vi "Sekvenser GFV.vi"(1 "Action(GET)":enum16{"GET", "SET"}(ring), 7 "Sequences":T1[](array[typedef]), 11 "error in (no error)":errorcluster) -> (8 "Sequences out":T1[](array[typedef]), 15 "error out":errorcluster)   [LabVIEW 2011]
uses:
  Complete sequence cluster holder.ctl
  User input.ctl
  Sequence steps config..ctl
  Single criteria cluster.ctl
  Criteria types.ctl
  Boolean operation.ctl
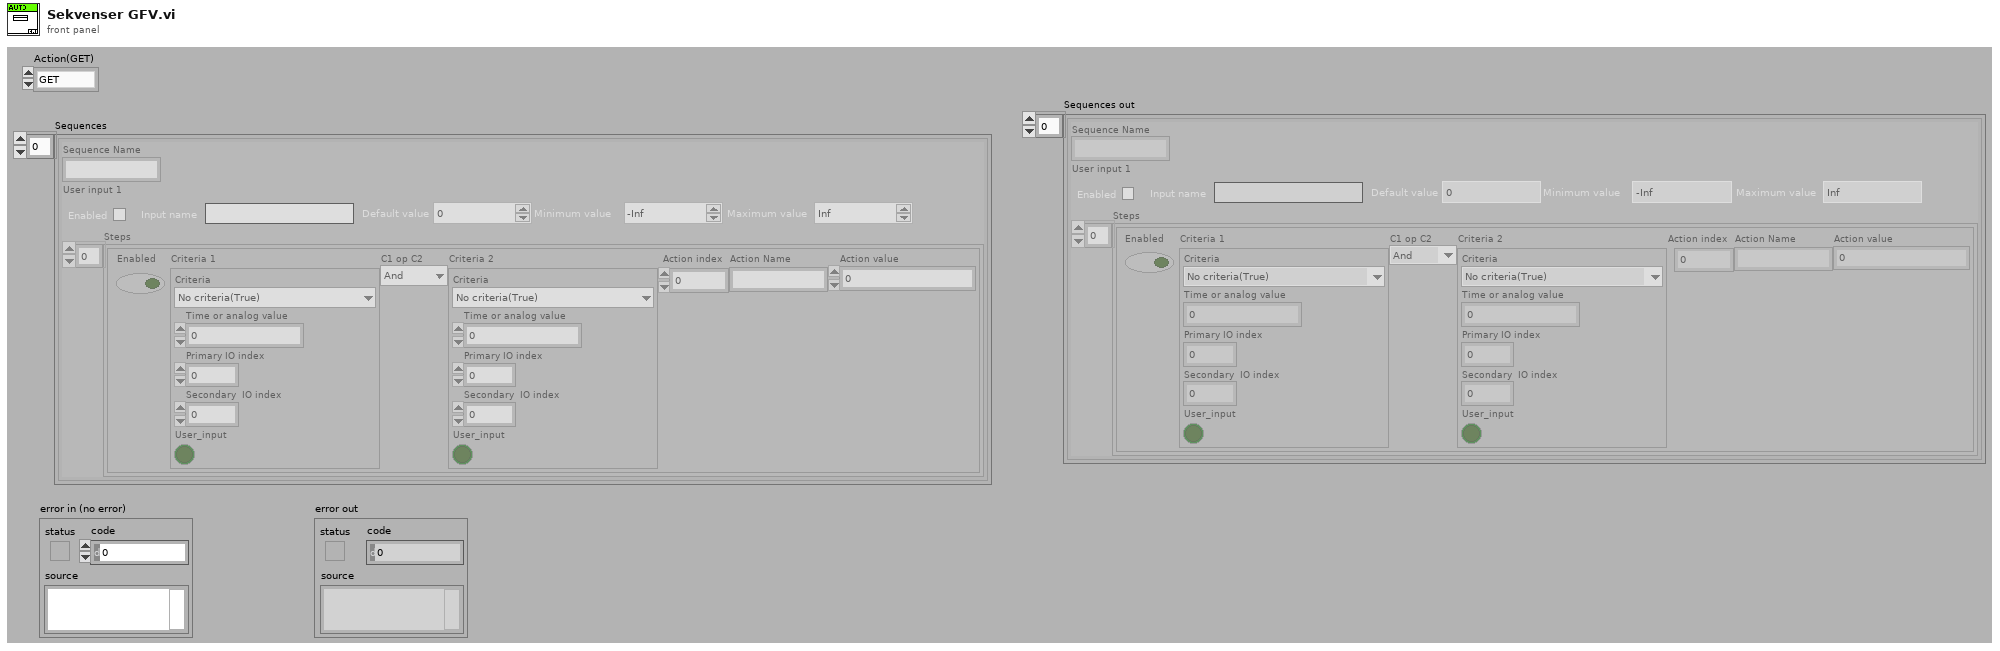
[diagram p1: front panel]
types:
  T1 = typedef "Complete sequence cluster holder.ctl" = cluster{"Sequence Name":string, "User input 1":T2, "Steps":T3[]}
  T2 = typedef "User input.ctl" = cluster{"Input name":string, "Minimum value ":dbl, "Maximum value":dbl, "Default value":dbl, "User inp enabled":bool}
  T3 = typedef "Sequence steps config..ctl" = cluster{"Enabled":bool, "Criteria 1":T4, "C1 op C2":T6, "Criteria 2":T4, "Action index":i32, "Action Name":string, "Action value":dbl}
  T4 = typedef "Single criteria cluster.ctl" = cluster{"Criteria":T5, "Time or analog value":dbl, "Primary IO index":i32, "Secondary  IO index":i32, "User_input":bool}
  T5 = typedef "Criteria types.ctl" = enum16{"No criteria(True)", "Time(s)", "Analog IO over", "Analog IO over or equal", "Analog IO under", "Analog IO under or equal", "Analog IO 1 minus Analog IO 2 over", "Digital IO True", "Digital IO False", "Operator approval"}
  T6 = typedef "Boolean operation.ctl" = enum16{"And", "Or", "Xor", "Nand", "Nor", "Nxor", "Implies"}
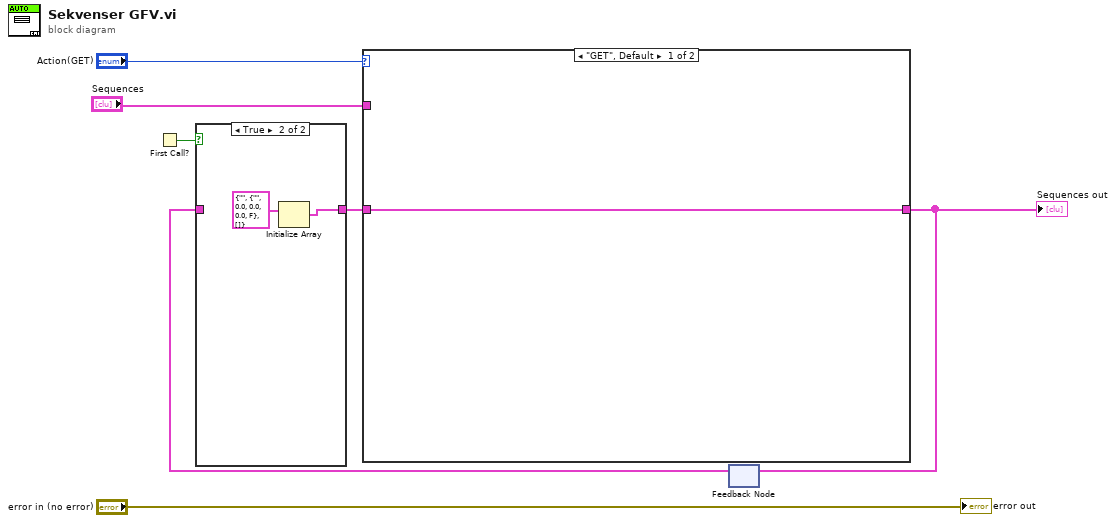
[diagram p0: block diagram]
diagram:
  n1 = First Call?() -> (First Call?: T/F=w4:bool)
  n2 = feedback #1() -> (w5:T1[])  [unwired: 1 in]
  n3 = case shown="True" w4 {
    tunnel: w5 -> [w8 _]
    tunnel: [w8 w9] -> w3
    frame False {
    }
    frame True {
      n4 = Initialize Array(T1 {"Sequence Name"="", "User input 1"={"Input name"="", "Minimum value "=0.0, "Maximum value"=0.0, "Default value"=0.0, "User inp enabled"=FALSE}, "Steps"=[]} ("Sequence")) -> (w9:T1[])  [unwired: 1 in]
    }
  }
  n5 = case shown="\"GET\", Default" "Action(GET)" {
    tunnel: [w11 w12] -> w2
    tunnel: w3 -> [w11 _]
    tunnel: "Sequences" -> [_ w12]
    frame "GET", Default {
    }
    frame "SET" {
    }
  }
  "Sequences out" <- w2
  n6 = feedback-in #1(w2) -> ()
  "error out" <- "error in (no error)"
